vi "DataConversion(SingleSample).vi"(2 "data":dbl[](array[numeric]), 3 "input cluster":T1, 4 "Init":bool=TRUE) -> (6 "Temperature":dbl, 7 "All Data":dbl[](array[numeric]), 8 "Red Data":dbl, 9 "Pressure":dbl, 10 "Blue Data":dbl)   [LabVIEW 2013, in "main.lvlib"]
uses:
  main.lvlib
  <vilib>/Analysis/3filter.llb/Filter Passband Type.ctl
  <vilib>/Analysis/3filter.llb/Filter Structure Type.ctl
  <vilib>/Analysis/NI_AALBase.lvlib
  <vilib>/ptbypt/NI_PtbyPt.lvlib
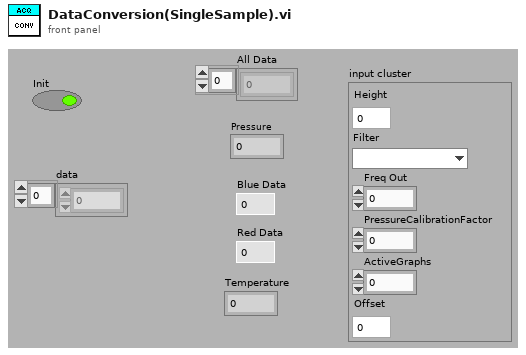
[diagram p1: front panel]
types:
  T1 = cluster{"Height":dbl, "Filter":u16, "Freq Out":i32, "PressureCalibrationFactor":dbl, "ActiveGraphs":u16, "Offset":dbl}
  T2 = typedef "NI_AALBase.lvlib/Filter Passband Type.ctl" = enum32{"Lowpass", "Highpass", "Bandpass", "Bandstop"}
  T3 = typedef "NI_AALBase.lvlib/Filter Structure Type.ctl" = u16
  T4 = cluster{"filter structure":enum32{"IIR 2nd Order", "IIR 4th Order"}, "Reverse Coefficients":dbl[], "Forward Coefficients":dbl[]}
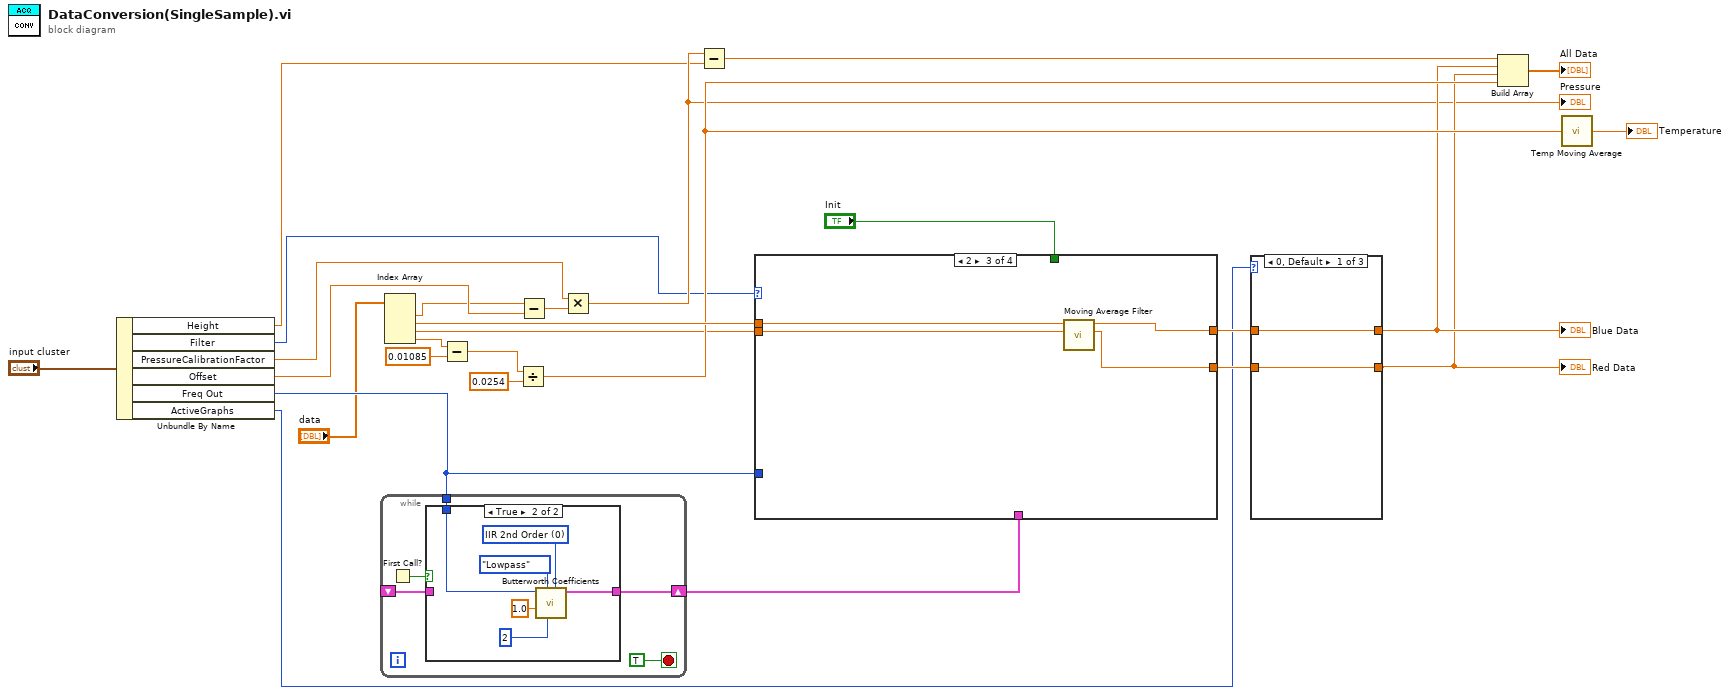
[diagram p0: block diagram]
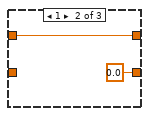
[diagram p3: hidden frame]
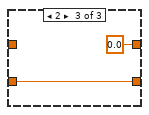
[diagram p4: hidden frame]
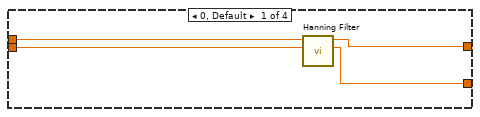
[diagram p5: hidden frame]
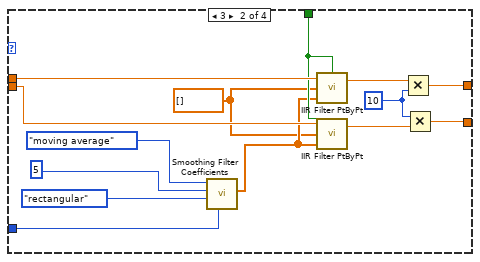
[diagram p6: hidden frame]
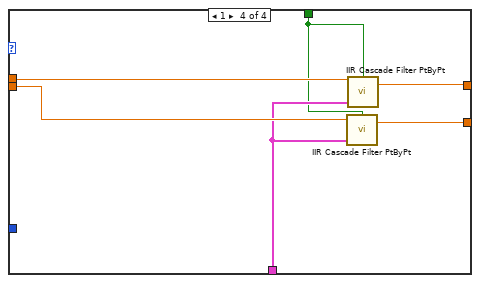
[diagram p7: hidden frame]
diagram:
  n1 = Unbundle By Name("input cluster") -> ("Height"=w3:dbl, "Filter"=w2:u16, "PressureCalibrationFactor"=w5:dbl, "Offset"=w8:dbl, "Freq Out"=w10:i32, "ActiveGraphs"=w9:u16)
  n2 = while {
    tunnel: w10 -> [w32]
    shift-right: [w30] -> w13
    shift-left: _ -> [w29]
    stop <- TRUE stop-if-true
    n3 = First Call?() -> (First Call?: T/F=w31:bool)
    n4 = case shown="True" w31 {
      tunnel: w32 -> [_ w39]
      tunnel: [w33 w34] -> w30
      tunnel: w29 -> [w33 _]
      frame False {
      }
      frame True {
        w37 = T3 0 items=["IIR 2nd Order"=0, "IIR 4th Order"=1, "Auto Select"=10] ("filter structure option")
        n5 = call <vilib>:"Butterworth Coefficients.vi"("filter structure option"=w37, "order"=2, "filter type"=Filter_Passband_Type."Lowpass", "low cutoff freq: fl"=1.0, "sampling freq: fs"=w39) -> ("IIR Filter Cluster"=w34:T4)  [unwired: 5 in, 1 out]
      }
    }
  }
  n6 = Index Array(array="data") -> (element #1=w7:dbl, element #2=w25:dbl, element #3=w12:dbl, element #4=w16:dbl)  [unwired: 4 in]
  n7 = Subtract(x=w16, y=0.01085) -> (x-y=w18:dbl)
  n8 = Divide(x=w18, y=0.0254 ("Temperature Sensitivity")) -> (x/y=w23:dbl)
  n9 = Subtract(x=w7, y=w8) -> (x-y=w6:dbl)
  n10 = Multiply(x=w5, y=w6) -> (x*y=w4:dbl)
  "Pressure" <- w4
  n11 = Subtract(x=w4, y=w3) -> (x-y=w24:dbl)
  n12 = case shown="2" w2 {
    tunnel: w12 -> [w42 w47 w60 w67]
    tunnel: w25 -> [w43 w54 w61 w64]
    tunnel: [w41 w51 w58 w65] -> w20
    tunnel: [w40 w46 w59 w66] -> w19
    tunnel: w10 -> [_ w53 _ _]
    tunnel: "Init" -> [_ w52 _ w62]
    tunnel: w13 -> [_ _ _ w63]
    frame 0, Default {
      n13 = call "Hanning Filter.vi"("Input 2"=w42, "Input"=w43) -> ("Filtered2"=w40:dbl, "Filtered"=w41:dbl)  [unwired: 8 in]
    }
    frame 3 {
      w44 = dbl[] []
      w48 = 10
      n14 = call <vilib>:"Smoothing Filter Coefficients.vi"("fs"=w53, "shape"=enum16{"rectangular", "triangular"}."rectangular", "half-width"=5, "type"=enum16{"moving average", "exponential"}."moving average") -> ("forward coefficients"=w45:dbl[])  [unwired: 5 in, 2 out]
      n15 = call <vilib>:"IIR Filter PtByPt.vi"("initialize"=w52, "Forward Coefficients"=w45, "Reverse Coefficients"=w44, "x"=w54) -> ("Filtered x"=w50:dbl)  [unwired: 1 out]
      n16 = call <vilib>:"IIR Filter PtByPt.vi"("initialize"=w52, "Forward Coefficients"=w45, "Reverse Coefficients"=w44, "x"=w47) -> ("Filtered x"=w49:dbl)  [unwired: 1 out]
      n17 = Multiply(x=w50, y=w48) -> (x*y=w51:dbl)
      n18 = Multiply(x=w48, y=w49) -> (x*y=w46:dbl)
    }
    frame 2 {
      n19 = call "Moving Average Filter.vi"("Input 2"=w60, "Input"=w61) -> ("Filtered2"=w59:dbl, "Filtered"=w58:dbl)  [unwired: 8 in]
    }
    frame 1 {
      n20 = call <vilib>:"IIR Cascade Filter PtByPt.vi"("initialize"=w62, "IIR Filter Cluster"=w63, "x"=w67) -> ("Filtered x"=w66:dbl)  [unwired: 1 in, 1 out]
      n21 = call <vilib>:"IIR Cascade Filter PtByPt.vi"("initialize"=w62, "IIR Filter Cluster"=w63, "x"=w64) -> ("Filtered x"=w65:dbl)  [unwired: 1 in, 1 out]
    }
  }
  n22 = case shown="0, Default" w9 {
    tunnel: [w69 w71 0.0 ("Filtered")] -> w15
    tunnel: w20 -> [w69 w71 _]
    tunnel: [w68 0.0 ("Filtered2") w73] -> w14
    tunnel: w19 -> [w68 _ w73]
    frame 0, Default {
    }
    frame 1 {
    }
    frame 2 {
    }
  }
  "Blue Data" <- w15
  "Red Data" <- w14
  n23 = Build Array(w24, w15, w14, w23) -> (→"All Data":dbl[])
  n24 = call "Temp Moving Average.vi"("PtByPt"=w23) -> ("Temperature"=→"Temperature":dbl)
